vi "边界检查器设定.vi"(0 "Image IN":T3(plugin-control), 1 "启动变量":bool, 2 "边界检查器参数":T2={"扇区个数"="1", "Fitted Circle (Find Circular Edge 1)"={"Center (Pixels)"={"X"=1736.0, "Y"=1501.0}, "Radius (Pixels)"=1442.0, "Center (Real-World)"={"X"=1736.0, "Y"=1501.0}, "Radius (Real-World)"=1442.0, "Roundness (Real-World)"=0.0, "Average Strength"=0.0, "Average SNR (dB)"=0.0}, "Range (Threshold 1)"={"Lower value"=65.0, "Upper value"=255.0}, "Process (Edge Detector 1)"=enum."Get All Edges", "Edge Options (Edge Detector 1)"={"Edge Polarity"=0, "Kernel Size"=9, "Width"=5, "Minimum Edge Strength"=27.0, "Interpolation Type"=enum."Bilinear", "Data Processing Method"=enum."Average"}} {"Edge Options (Edge Detector 1)"."Edge Polarity" items=["All Edges", "Rising Edges", "Falling Edges"]; "Fitted Circle (Find Circular Edge 1)"."Average SNR (dB)" format="%.2f"; "Fitted Circle (Find Circular Edge 1)"."Average Strength" format="%.2f"; "Fitted Circle (Find Circular Edge 1)"."Roundness (Real-World)" format="%.2f"; "Fitted Circle (Find Circular Edge 1)"."Radius (Real-World)" format="%.2f"; "Fitted Circle (Find Circular Edge 1)"."Center (Real-World)"."Y" format="%.2f"; "Fitted Circle (Find Circular Edge 1)"."Center (Real-World)"."X" format="%.2f"; "Fitted Circle (Find Circular Edge 1)"."Radius (Pixels)" format="%.2f"; "Fitted Circle (Find Circular Edge 1)"."Center (Pixels)"."Y" format="%.2f"; "Fitted Circle (Find Circular Edge 1)"."Center (Pixels)"."X" format="%.2f"}, 5 "error in":errorcluster) -> (14 "Image Out":T3(plugin-control), 15 "起始点":cluster{"X":sgl, "Y":sgl}[](array[cluster]), 16 "结束点":cluster{"X":sgl, "Y":sgl}[](array[cluster]), 17 "厚度":sgl[](array[numeric]), 19 "error out":errorcluster)   [LabVIEW 2017]
uses:
  <vilib>/vision/Measure.llb/Edge New.ctl
  Global System.vi
  <vilib>/vision/NI_Vision_Development_Module.lvlib
panel:
  out "millisecond timer value":u32
  out "Distances":sgl[](array[numeric]) format="%.4f"
  out "Edge Information (Edge Detector 1) 2":T1[](array[typedef]) {"Distance (Real-World)" format="%.2f"; "Location (Real-World)"."Y" format="%.2g"; "Location (Real-World)"."X" format="%.2f"; "Noise" format="%.2f"; "Location (Pixel)"."Y" format="%.2g"; "Location (Pixel)"."X" format="%.2f"; "Strength" format="%.2f"; "Distance (Pixel)" format="%.2f"}
  out "Edge Information (Edge Detector 1)":T1[][](array[typedef]) {"Distance (Real-World)" format="%.2f"; "Location (Real-World)"."Y" format="%.2g"; "Location (Real-World)"."X" format="%.2f"; "Noise" format="%.2f"; "Location (Pixel)"."Y" format="%.2g"; "Location (Pixel)"."X" format="%.2f"; "Strength" format="%.2f"; "Distance (Pixel)" format="%.2f"}
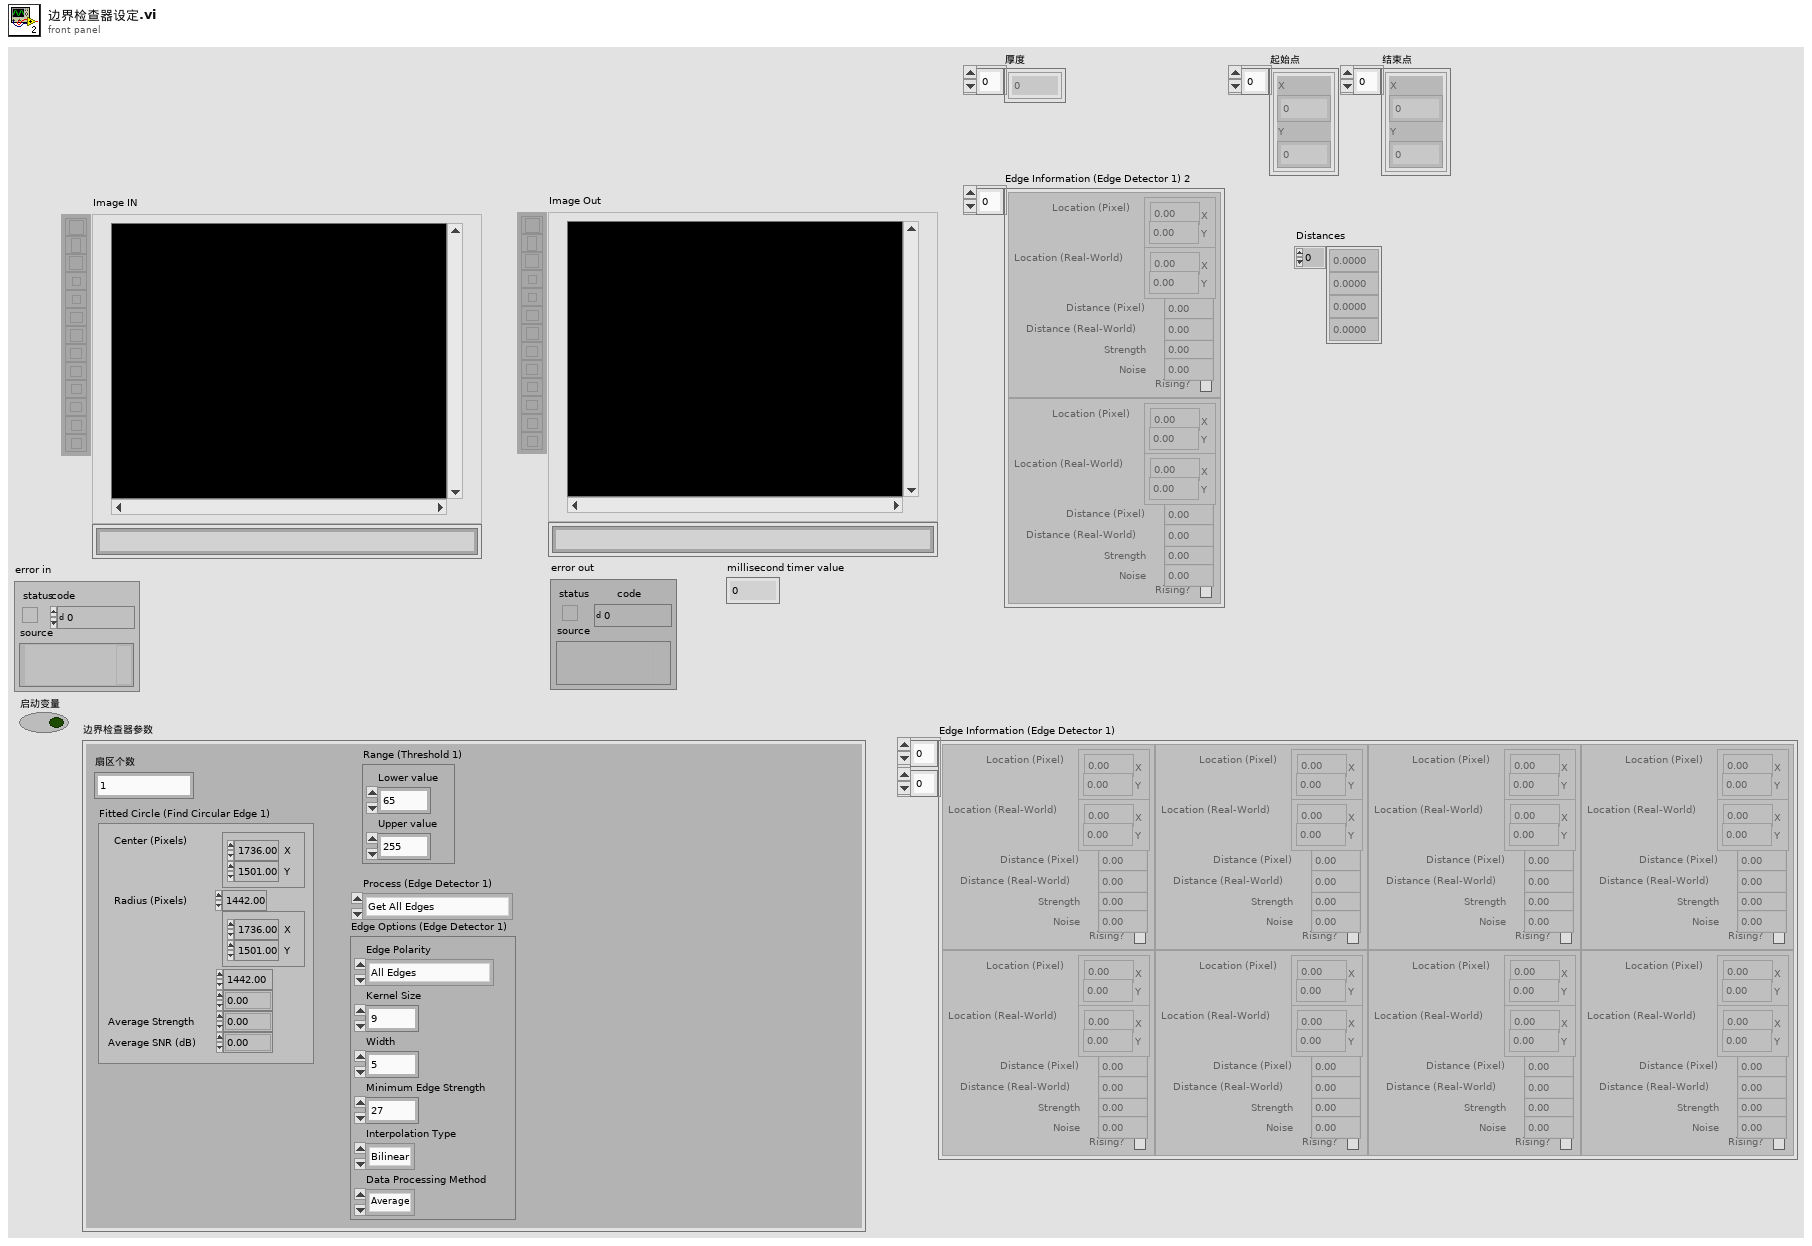
[diagram p1: front panel]
types:
  T1 = typedef "Edge New.ctl" = cluster{"Location (Pixel)":cluster{"X":sgl, "Y":sgl}, "Location (Real-World)":cluster{"X":sgl, "Y":sgl}, "Distance (Pixel)":dbl, "Distance (Real-World)":dbl, "Strength":dbl, "Noise":dbl, "Rising?":bool}
  T2 = cluster{"扇区个数":string, "Fitted Circle (Find Circular Edge 1)":cluster{"Center (Pixels)":cluster{"X":sgl, "Y":sgl}, "Radius (Pixels)":dbl, "Center (Real-World)":cluster{"X":sgl, "Y":sgl}, "Radius (Real-World)":dbl, "Roundness (Real-World)":dbl, "Average Strength":dbl, "Average SNR (dB)":dbl}, "Range (Threshold 1)":cluster{"Lower value":sgl, "Upper value":sgl}, "Process (Edge Detector 1)":enum16{"Get First Edge", "Get First + Last Edge", "Get All Edges", "Get Best Edge"}, "Edge Options (Edge Detector 1)":cluster{"Edge Polarity":u32, "Kernel Size":u32, "Width":u32, "Minimum Edge Strength":sgl, "Interpolation Type":enum32{"Zero Order", "Bilinear", "Quadratic", "Cubic", "Bilinear Fixed"}, "Data Processing Method":enum32{"Average", "Median"}}}
  T3 = typedef "IMAQ Image.ctl" = refnum<image>
  T4 = cluster{"Center (Pixels)":cluster{"X":sgl, "Y":sgl}, "Radius (Pixels)":dbl, "Center (Real-World)":cluster{"X":sgl, "Y":sgl}, "Radius (Real-World)":dbl, "Roundness (Real-World)":dbl, "Average Strength":dbl, "Average SNR (dB)":dbl}
  T5 = enum16{"Get First Edge", "Get First + Last Edge", "Get All Edges", "Get Best Edge"}
  T6 = cluster{"Edge Polarity":u32, "Kernel Size":u32, "Width":u32, "Minimum Edge Strength":sgl, "Interpolation Type":enum32{"Zero Order", "Bilinear", "Quadratic", "Cubic", "Bilinear Fixed"}, "Data Processing Method":enum32{"Average", "Median"}}
  T7 = typedef "IMAQ Line" = cluster{"Start X":i32, "Start Y":i32, "End X":i32, "End Y":i32}
  T8 = typedef "ROI Descriptor" = cluster{"Global Rectangle":i32[], "Contours":cluster{"ID":enum32{"External", "Internal"}, "Type":u32, "Coordinates":i32[]}[]}
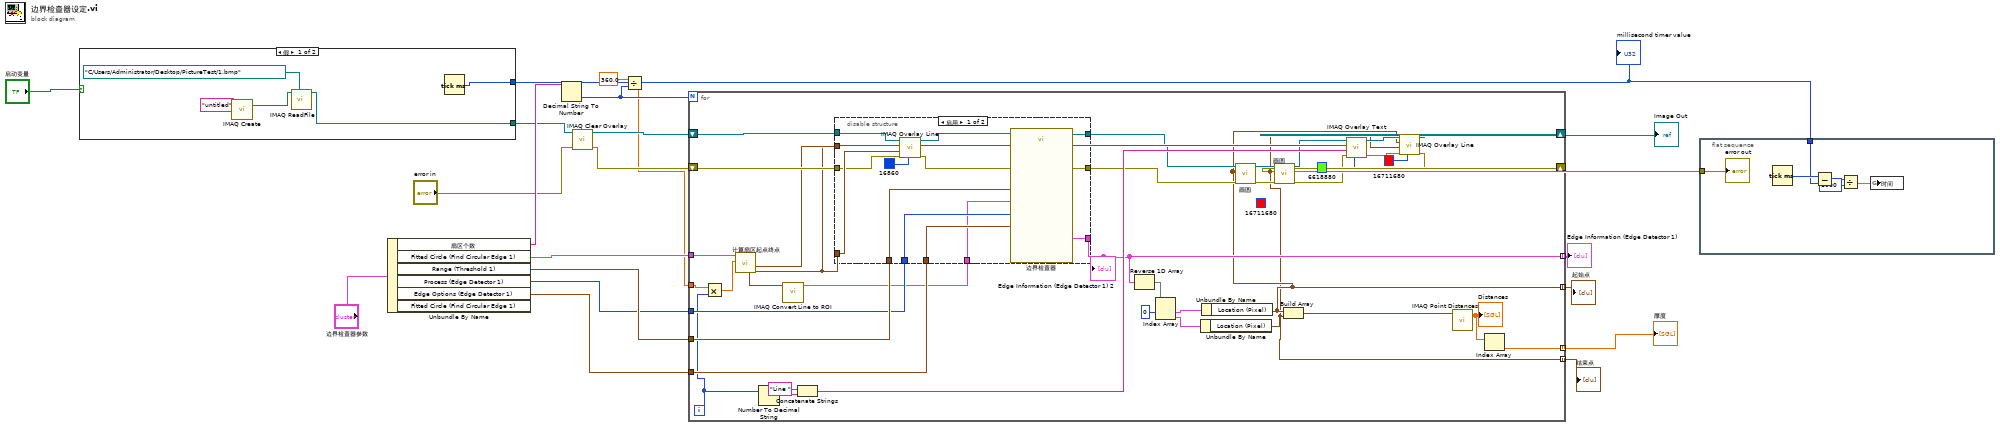
[diagram p0: block diagram]
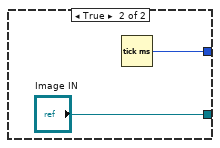
[diagram p2: hidden frame]
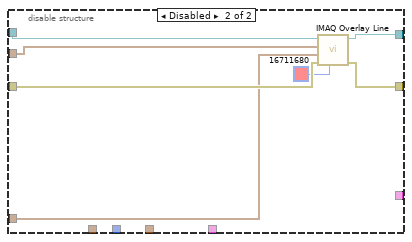
[diagram p3: hidden frame]
diagram:
  n1 = case shown="假" "启动变量" {
    tunnel: [w23 "Image IN"] -> w14
    tunnel: [w22 w27] -> w1
    frame False {
      n2 = call "IMAQ Create"("Image Name"="untitled") -> ("New Image"=w25:T3)  [unwired: 4 in, 1 out]
      n3 = call "IMAQ ReadFile"("File Path"=path "C:/Users/Administrator/Desktop/PictureTest/1.bmp", "Image"=w25) -> ("Image Out"=w23:T3)  [unwired: 5 in, 4 out]
      n4 = Tick Count (ms)() -> (millisecond timer value=w22:u32)
    }
    frame True {
      n5 = Tick Count (ms)() -> (millisecond timer value=w27:u32)
    }
  }
  "millisecond timer value" <- w1
  n6 = Unbundle By Name("边界检查器参数") -> ("扇区个数"=w18:string, "Fitted Circle (Find Circular Edge 1)"=w17:T4, "Range (Threshold 1)"=w10:cluster{"Lower value":sgl, "Upper value":sgl}, "Process (Edge Detector 1)"=w9:T5, "Edge Options (Edge Detector 1)"=w8:T6)  [unwired: 1 out]
  n7 = Decimal String To Number(string=w18) -> (number=w3:i32)  [unwired: 2 in, 1 out]
  n8 = call "IMAQ Clear Overlay"("error in (no error)"="error in", "Image"=w14) -> ("error out"=w11:errorcluster, "Image Out"=w13:T3)  [unwired: 8 in]
  n9 = Divide(x=360.0, y=w3) -> (x/y=w2:dbl)
  n10 = for {
    N: w3 -> [_]
    shift-right: [w34] -> w21
    shift-left: w13 -> [w66]
    shift-right: [w32] -> w20
    shift-left: w11 -> [w65]
    tunnel: w17 -> [w64]
    tunnel: w2 -> [w62]
    tunnel: w10 -> [w60]
    tunnel: w9 -> [w59]
    tunnel: w8 -> [w58]
    tunnel: [w37] -> w7 mode=indexing
    tunnel: [w31] -> w6 mode=indexing
    tunnel: [w30] -> w5 mode=indexing
    tunnel: [w50] -> w4 mode=indexing
    i -> [w49]
    (unwired) u32 16711680 ("Color")
    n11 = Multiply(x=w62, y=w49) -> (x*y=w61:dbl)
    n12 = call "计算扇区起点终点.vi"("角度"=w61, "Fitted Circle (Find Circular Edge 1)"=w64) -> ("EndPos"=w44:cluster{"dx":dbl, "dy":dbl}, "StartPos"=w63:cluster{"X":sgl, "Y":sgl}, "输出簇"=w57:T7)  [unwired: 5 in, 2 out]
    n13 = Number To Decimal String(number=w49) -> (decimal integer string=w47:string)  [unwired: 1 in]
    n14 = call "IMAQ Convert Line to ROI"("Line"=w57) -> ("ROI Descriptor"=w56:T8)  [unwired: 8 in, 1 out]
    n15 = Concatenate Strings("Line " ("字符串"), w47) -> (w46:string)
    n16 = disable-structure shown="启用" {
      disable-tunnel: w66 -> [w72 w87]
      disable-tunnel: [w80 w86] -> w43
      disable-tunnel: w65 -> [w68 w84]
      disable-tunnel: [w79 w85] -> w40
      disable-tunnel: w63 -> [w70 w82]
      disable-tunnel: w44 -> [w69 w81]
      disable-tunnel: w60 -> [w78 _]
      disable-tunnel: w59 -> [w77 _]
      disable-tunnel: w58 -> [w76 _]
      disable-tunnel: w56 -> [w75 _]
      disable-tunnel: [w74 _] -> w37
      frame Enabled {
        n17 = call "IMAQ Overlay Line"("Color"=u32 16860, "error in (no error)"=w68, "End Point"=w69, "Start Point"=w70, "Image"=w72) -> ("error out"=w67:errorcluster, "Image Out"=w71:T3)  [unwired: 5 in]
        n18 = call "边界检查器"("Image In"=w71, "Range (Threshold 1)"=w78, "ROI Descriptor (Edge Detector 1)"=w75, "Process (Edge Detector 1)"=w77, "Edge Options (Edge Detector 1)"=w76, "error in"=w67) -> ("Image Out"=w80:T3, "Edge Information (Edge Detector 1)"=w74:T1[], "error out"=w79:errorcluster)  [unwired: 19 in]
      }
      frame Disabled {
        n19 = call "IMAQ Overlay Line"("Color"=u32 16711680, "error in (no error)"=w84, "End Point"=w81, "Start Point"=w82, "Image"=w87) -> ("error out"=w85:errorcluster, "Image Out"=w86:T3)  [unwired: 5 in]
      }
    }
    "Edge Information (Edge Detector 1) 2" <- w37
    n20 = Reverse 1D Array(array=w37) -> (reversed array=w36:T1[])
    n21 = Index Array(array=w36, index #1=0 ("索引")) -> (element #1=w54:T1, element #2=w53:T1)  [unwired: 1 in]
    n22 = Unbundle By Name(w53) -> ("Location (Pixel)"=w30:cluster{"X":sgl, "Y":sgl})
    n23 = Unbundle By Name(w54) -> ("Location (Pixel)"=w31:cluster{"X":sgl, "Y":sgl})
    n24 = call "画圆.vi"("error in (no error)"=w40, "Location (Pixel)"=w31, "Image in"=w43) -> ("error out"=w39:errorcluster, "Image out"=w42:T3)  [unwired: 7 in]
    n25 = call "画圆.vi"("error in (no error)"=w39, "Location (Pixel)"=w30, "Image in"=w42) -> ("error out"=w38:errorcluster, "Image out"=w41:T3)  [unwired: 7 in]
    n26 = Build Array(w31, w30) -> (w52:cluster{"X":sgl, "Y":sgl}[])
    n27 = call "IMAQ Overlay Text"("Text Color (black)"=u32 6618880, "error in (no error)"=w38, "String"=w46, "Origin"=w44, "Image"=w41) -> ("error out"=w33:errorcluster, "Image Out"=w35:T3)  [unwired: 5 in]
    n28 = call "IMAQ Overlay Line"("Color"=u32 16711680, "error in (no error)"=w33, "End Point"=w30, "Start Point"=w31, "Image"=w35) -> ("error out"=w32:errorcluster, "Image Out"=w34:T3)  [unwired: 5 in]
    n29 = call "IMAQ Point Distances"("Points"=w52) -> ("Distances"=w51:sgl[])  [unwired: 4 in, 1 out]
    "Distances" <- w51
    n30 = Index Array(array=w51) -> (element=w50:sgl)  [unwired: 1 in]
  }
  "Image Out" <- w21
  "Edge Information (Edge Detector 1)" <- w7
  "起始点" <- w6
  "结束点" <- w5
  "厚度" <- w4
  n31 = flat-sequence {
    tunnel: w20 -> [w93]
    tunnel: w1 -> [w91]
    frame #0 {
      n32 = Tick Count (ms)() -> (millisecond timer value=w92:u32)
      n33 = Subtract(x=w92, y=w91) -> (x-y=w90:u32)
      n34 = Divide(x=w90, y=u32 1000) -> (x/y=w88:dbl)
      n35 = global write "Global System.vi" "时间"(w88) -> ()
      "error out" <- w93
    }
  }
